vi "Save DAC Configuration.vi"(8 "error in":errorcluster, 10 "Config File refnum in":T1, 11 "DAC Jumo DP in":refnum<class "DAC Jumo DP.lvclass">) -> (0 "error out":errorcluster, 2 "Config File refnum out":T1, 3 "DAC Jumo DP out":refnum<class "DAC Jumo DP.lvclass">)   [LabVIEW 2019, in "DAC.lvlib" / "DAC Jumo DP.lvclass"]
uses:
  DAC Jumo DP.lvclass
  C:/Users/wg/Documents/LV_Projects/test-stand/App/DAC/DAC.lvclass
  <vilib>/Utility/config.llb/Config Data RefNum.ctl
  DAC.lvclass/DAC.ctl
  DAC Jumo DP.lvclass/DAC Jumo DP.ctl
  <vilib>/Utility/config.llb/Write Key (String).vi
  DAC.lvclass
  <vilib>/Utility/config.llb/NI_LVConfig.lvlib
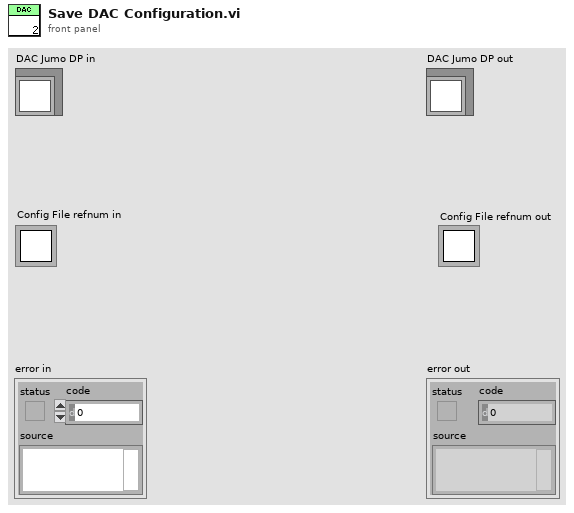
[diagram p1: front panel]
types:
  T1 = typedef "NI_LVConfig.lvlib/Config Data RefNum.ctl" = refnum<k1>
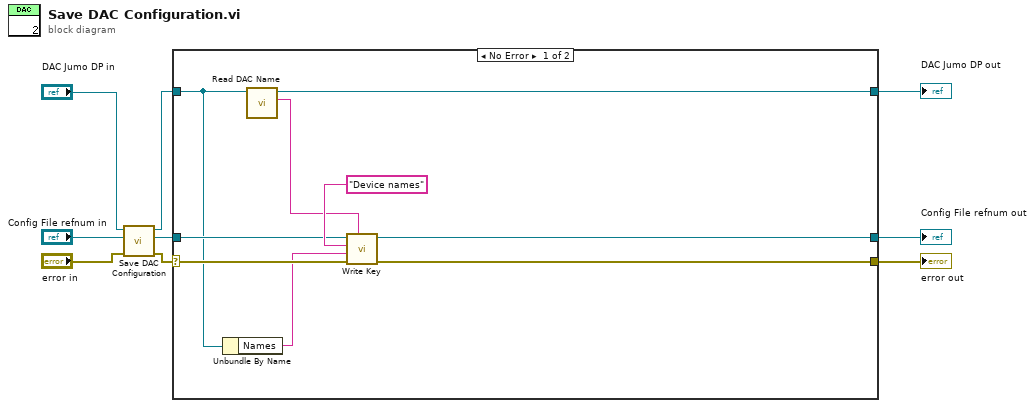
[diagram p0: block diagram]
diagram:
  n1 = call-parent "Save DAC Configuration.vi"("error in"="error in", "Config File refnum in"="Config File refnum in", "DAC in"="DAC Jumo DP in") -> ("error out"=w4:errorcluster, "Config File refnum out"=w5:T1, "DAC out"=w6:refnum<class "DAC Jumo DP.lvclass">)  [unwired: 6 in]
  n2 = case shown="No Error" w4 {
    selector: w4 -> [w16 w21]
    tunnel: [w10 w21] -> w1
    tunnel: [w14 w20] -> w3
    tunnel: w6 -> [w15 w20]
    tunnel: w5 -> [w17 w19]
    tunnel: [w11 w19] -> w2
    frame No Error {
      n3 = Unbundle By Name(w15) -> ("Names"=w12:string)
      n4 = call "Read DAC Name.vi"("DAC in"=w15) -> ("DAC Name"=w13:string, "DAC out"=w14:refnum<class "DAC Jumo DP.lvclass">)  [unwired: 8 in, 1 out]
      n5 = call-poly <vilib>:"Write Key.vi"("section"=w13, "error in (no error)"=w16, "value"=w12, "key"="Device names", "refnum"=w17) -> ("error out"=w10:errorcluster, "refnum out"=w11:T1)  [unwired: 4 in, 1 out]
    }
    frame Error {
    }
  }
  "error out" <- w1
  "DAC Jumo DP out" <- w3
  "Config File refnum out" <- w2
